vi "Score Event Refnum.vi"() -> ()   [LabVIEW 2013]
panel:
  in  "user event out":refnum<user-event>
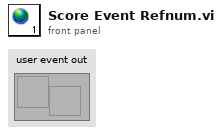
[diagram p1: front panel]
diagram:
